vi "Convert Material JSON to LabVIEW Theme.vi"() -> ()   [LabVIEW 2021]
doc: "Convert existing material3 json files exported from Google to be used with TSC Material application VIs.\n\n<b>Code Developed By:</b>\nDaniel Coons\nTechnology Service Corporation\nwww.tsc.com/atcs"
uses:
  Material Theme/Material Theme.lvclass
  <vilib>/Utility/traverseref.llb/TRef TravTarget.ctl
  _Material Theme SubVIs/material theme.ctl
  _Material Theme SubVIs/material json scheme.ctl
  _Material Theme SubVIs/material json palette.ctl
  Material-Scheme/Material-Scheme.lvclass/Material-Scheme.ctl
  8aff6bdd-0f42-4725-a4f4-6aecb987c99b.vi
  Material-Scheme/data member access/get surface.vi
  Material-Scheme/data member access/Read name.vi
  <vilib>/JDP Science/JSONtext/JSON text to Variant.vi
  <vilib>/JDP Science/JSONtext/LVClass Serializer/JSONtext LVClass Serializer.lvclass
  Material-Palette/Material-Palette.lvclass
  Material-Scheme/Material-Scheme.lvclass
  user32.dll
  <vilib>/Utility/traverseref.llb/VI Scripting - Traverse.lvlib
panel:
  in  "tabs":enum32{"color", "palette", "json"}(radio)
  in  "preview":bool
  in  "close":bool
  out "header":bool
  in  "save":bool
  in  "Theme":u16(ring) items=["Light Theme", "Light Medium Contrast", "Light High Contrast", "Dark Theme", "Dark Medium Contrast", "Dark High Constrast"]
  in  "Tab Control":T1(tab)
  out "material JSON output":string
  in  "file path":path
  # "Convert a JSON M3 theme file from Google to use the TSC Material Theme in a VI"
  # "Can be generated through Figma or at:   https://material-foundation.github.io/material-theme-builder/<Material Website>"
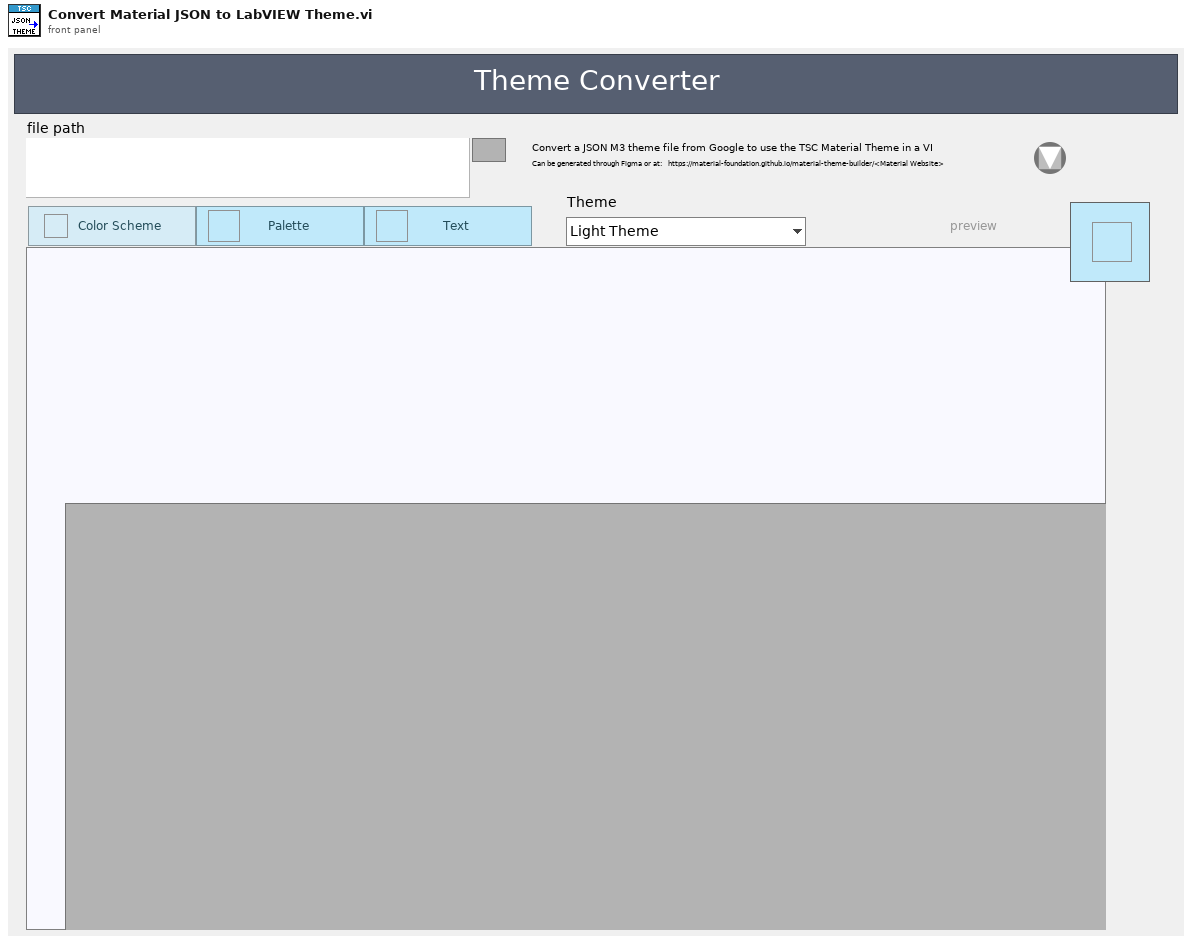
[diagram p1: front panel]
types:
  T1 = enum32{"Color Scheme", "Palette Variations", "JSON String"}
  T2 = typedef "TRef TravTarget.ctl" = enum16{"FP", "BD", "Other"}
  T3 = typedef "material theme.ctl" = cluster{"description":string, "seed":string, "coreColors":cluster{"primary":string, "secondary":string, "tertiary":string, "error":string}, "schemes":cluster{"light":T4, "light-medium-contrast":T4, "light-high-contrast":T4, "dark":T4, "dark-medium-contrast":T4, "dark-high-contrast":T4}, "palettes":cluster{"primary":T5, "secondary":T5, "tertiary":T5, "neutral":T5, "neutral-variant":T5}}
  T4 = typedef "material json scheme.ctl" = cluster{"primary":string, "surfaceTint":string, "onPrimary":string, "primaryContainer":string, "onPrimaryContainer":string, "secondary":string, "onSecondary":string, "secondaryContainer":string, "onSecondaryContainer":string, "tertiary":string, "onTertiary":string, "tertiaryContainer":string, "onTertiaryContainer":string, "error":string, "onError":string, "errorContainer":string, "onErrorContainer":string, "background":string, "onBackground":string, "surface":string, "onSurface":string, "surfaceVariant":string, "onSurfaceVariant":string, "outline":string, "outlineVariant":string, "shadow":string, "scrim":string, "inverseSurface":string, "inverseOnSurface":string, "inversePrimary":string, "primaryFixed":string, "onPrimaryFixed":string, "primaryFixedDim":string, "onPrimaryFixedVariant":string, "secondaryFixed":string, "onSecondaryFixed":string, "secondaryFixedDim":string, "onSecondaryFixedVariant":string, "tertiaryFixed":string, "onTertiaryFixed":string, "tertiaryFixedDim":string, "onTertiaryFixedVariant":string, "surfaceDim":string, "surfaceBright":string, "surfaceContainerLowest":string, "surfaceContainerLow":string, "surfaceContainer":string, "surfaceContainerHigh":string, "surfaceContainerHighest":string}
  T5 = typedef "material json palette.ctl" = cluster{"0":string, "5":string, "10":string, "15":string, "20":string, "25":string, "30":string, "35":string, "40":string, "50":string, "60":string, "70":string, "80":string, "90":string, "95":string, "98":string, "99":string, "100":string}
  T6 = enum16{"open", "replace", "create", "open or create", "replace or create", "replace or create with confirmation"}
  T7 = typedef "LVRectTypeDef.ctl" = cluster{"Left":i16, "Top":i16, "Right":i16, "Bottom":i16}
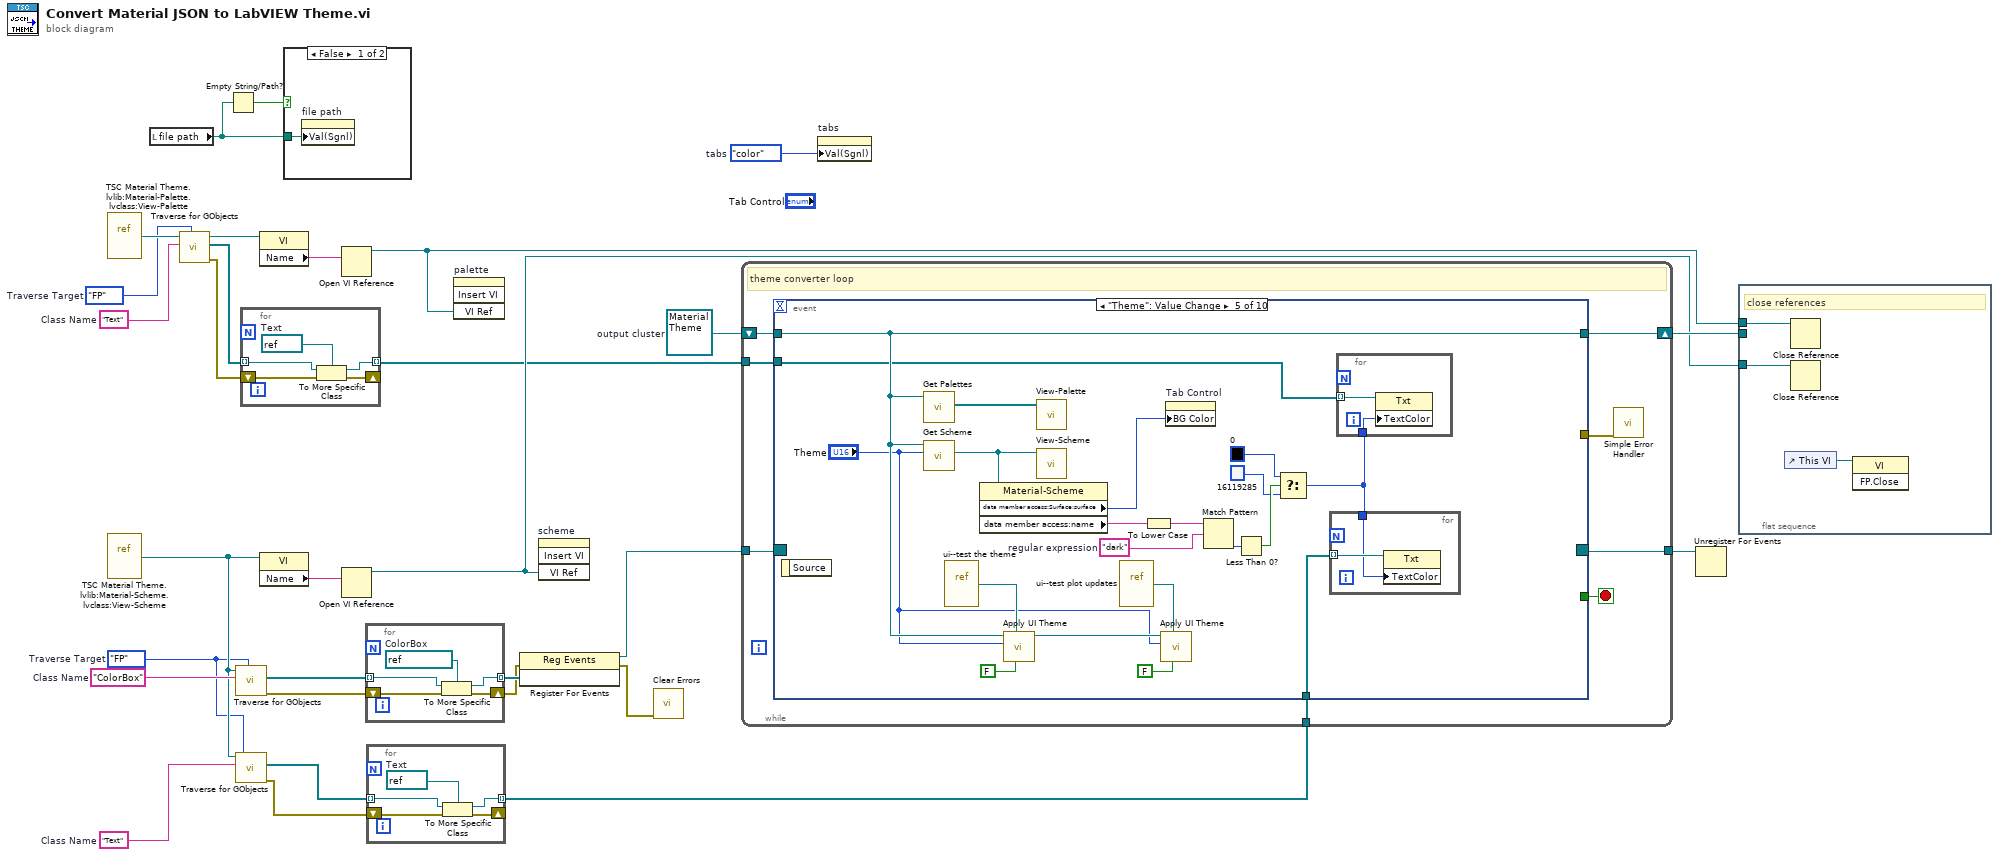
[diagram p0: block diagram]
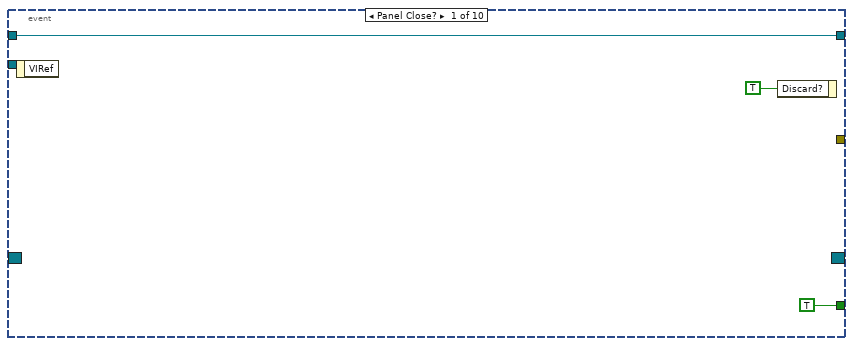
[diagram p3: hidden frame]
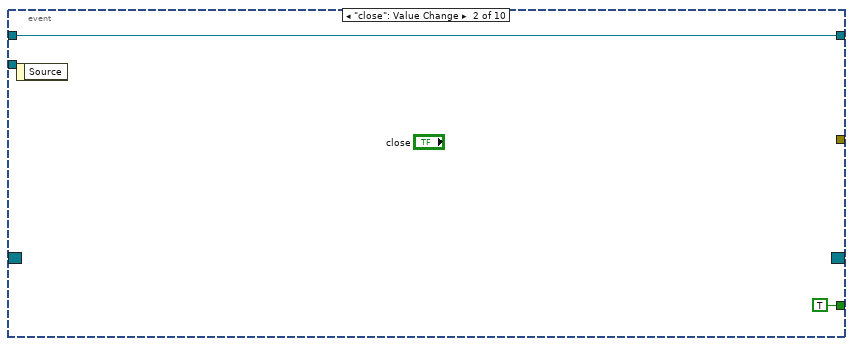
[diagram p4: hidden frame]
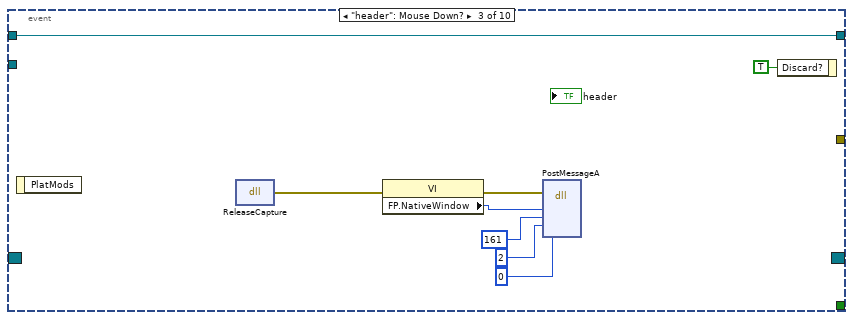
[diagram p5: hidden frame]
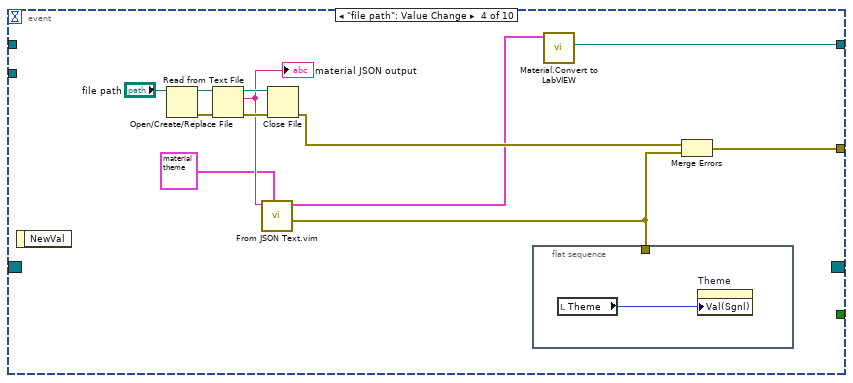
[diagram p6: hidden frame]
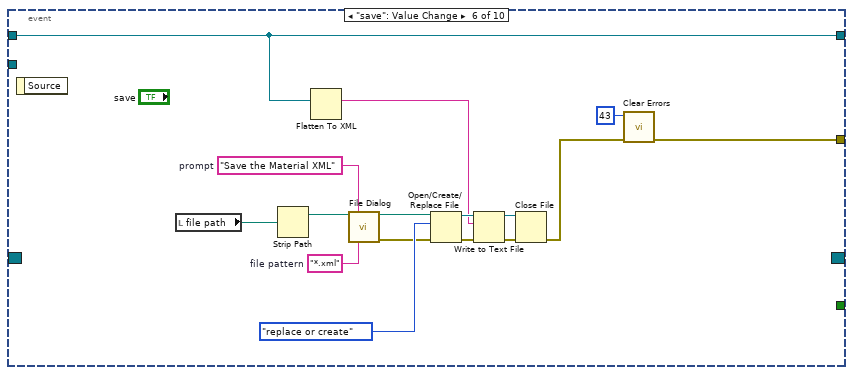
[diagram p7: hidden frame]
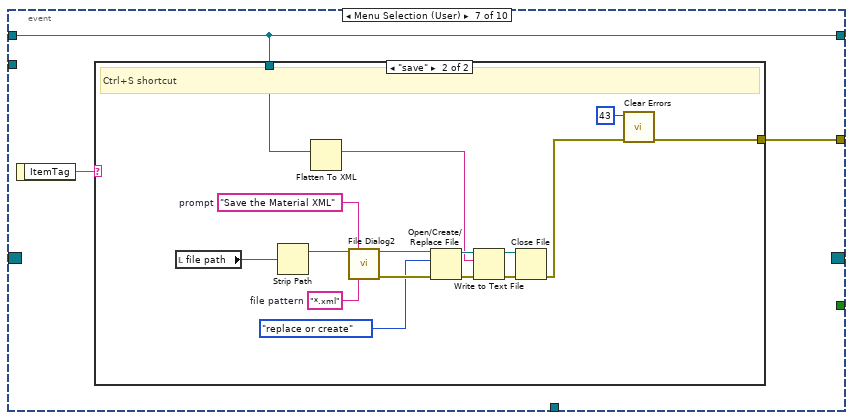
[diagram p8: hidden frame]
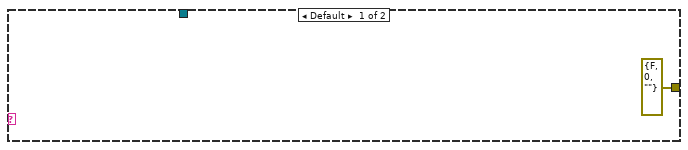
[diagram p9: hidden frame]
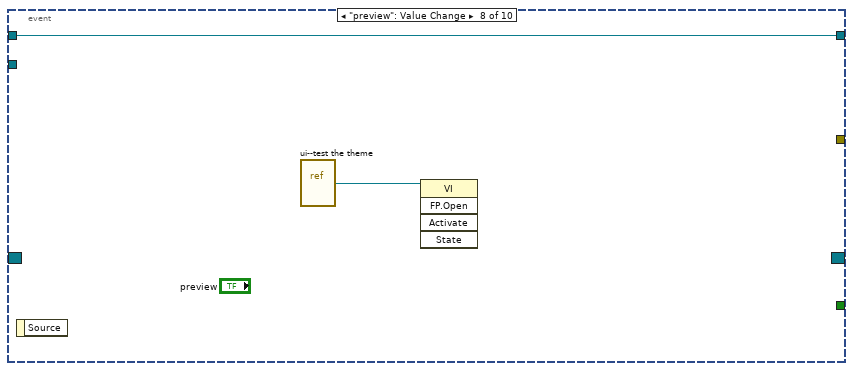
[diagram p10: hidden frame]
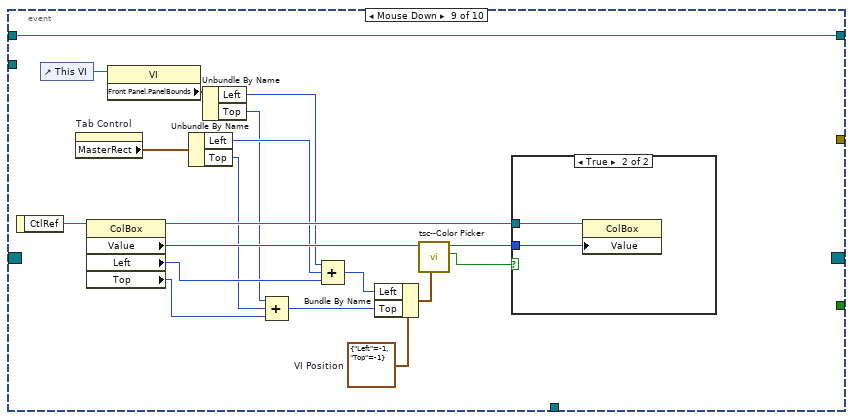
[diagram p11: hidden frame]
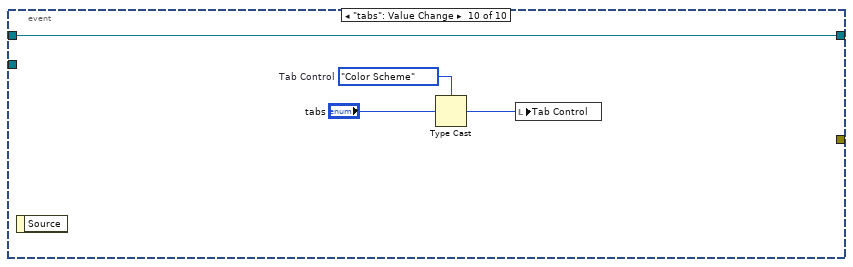
[diagram p13: hidden frame]
diagram:
  w6 = "Text"  # Class Name
  w10 = "Text"  # Class Name
  w11 = TRef_TravTarget."FP"  # Traverse Target
  w13 = enum32{"color", "palette", "json"}."color"  # tabs
  w16 = refnum<class "Material Theme.lvclass"> refnum  # output cluster
  w25 = "ColorBox"  # Class Name
  w4 = TRef_TravTarget."FP"  # Traverse Target
  n1 = vi-ref "TSC Material Theme.lvlib:Material-Palette.lvclass:View-Palette.vi"() -> (w30:refnum<vi>)
  n2 = vi-ref "TSC Material Theme.lvlib:Material-Scheme.lvclass:View-Scheme.vi"() -> (w5:refnum<vi>)
  n3 = local read "file path"() -> (w15:path)
  n4 = call <vilib>:"Traverse for GObjects.vi"("Traverse Target"=w11, "Class Name"=w10, "VI Refnum"=w30) -> ("error out"=w7:errorcluster, "References"=w9:refnum<vi>[], "dup VI Refnum"=w12:refnum<vi>)  [unwired: 5 in, 1 out]
  n5 = Empty String/Path?(string/path=w15) -> (empty?=w14:bool)
  n6 = call <vilib>:"Traverse for GObjects.vi"("Traverse Target"=w4, "Class Name"=w25, "VI Refnum"=w5) -> ("error out"=w19:errorcluster, "References"=w23:refnum<vi>[])  [unwired: 5 in, 2 out]
  n7 = call <vilib>:"Traverse for GObjects.vi"("Traverse Target"=w4, "Class Name"=w6, "VI Refnum"=w5) -> ("error out"=w2:errorcluster, "References"=w3:refnum<vi>[])  [unwired: 5 in, 2 out]
  n8 = for {
    tunnel: w9 -> [w32] mode=indexing
    shift-right: [w34] -> _
    shift-left: w7 -> [w35]
    tunnel: [w31] -> w8 mode=indexing
    w33 = refnum<vi> refnum  # Text
    n9 = To More Specific Class(target class=w33, reference=w32, error in=w35) -> (specific class reference=w31:refnum<vi>, error out=w34:errorcluster)
  }
  n10 = property class="VI"(reference=w12) -> ("Name"=w29:string)  [unwired: 1 in, 2 out]
  n11 = property class="VI"(reference=w5) -> ("Name"=w28:string)  [unwired: 1 in, 2 out]
  n12 = case shown="False" w14 {
    tunnel: w15 -> [w36 _]
    frame False {
      n13 = property on="file path" class="Path"("Val(Sgnl)"=w36) -> ()  [unwired: 2 in, 2 out]
    }
    frame True {
    }
  }
  n14 = Open VI Reference(vi path=w29) -> (vi reference=w26:refnum<vi>)  [unwired: 5 in, 1 out]
  n15 = Open VI Reference(vi path=w28) -> (vi reference=w22:refnum<vi>)  [unwired: 5 in, 1 out]
  n16 = for {
    tunnel: w23 -> [w38] mode=indexing
    shift-right: [w40] -> w18
    shift-left: w19 -> [w41]
    tunnel: [w37] -> w21 mode=indexing
    w39 = refnum<vi> refnum  # ColorBox
    n17 = To More Specific Class(target class=w39, reference=w38, error in=w41) -> (specific class reference=w37:refnum<vi>, error out=w40:errorcluster)
  }
  n18 = for {
    tunnel: w3 -> [w43] mode=indexing
    shift-right: [w45] -> _
    shift-left: w2 -> [w46]
    tunnel: [w42] -> w1 mode=indexing
    w44 = refnum<vi> refnum  # Text
    n19 = To More Specific Class(target class=w44, reference=w43, error in=w46) -> (specific class reference=w42:refnum<vi>, error out=w45:errorcluster)
  }
  n20 = invoke on="palette" class="SubPnl" method="Insert VI"("VI Ref"=w26) -> ()  [unwired: 3 in, 4 out]
  n21 = register-events(error in=w18, w21) -> (reference out=w24:refnum<event-registration>, error out=w17:errorcluster)  [unwired: 1 in]
  n22 = invoke on="scheme" class="SubPnl" method="Insert VI"("VI Ref"=w22) -> ()  [unwired: 3 in, 4 out]
  n23 = call <vilib>:"Clear Errors.vi"("error in (no error)"=w17) -> ()  [unwired: 5 in, 2 out]
  n24 = while {
    shift-right: [w53] -> w27
    shift-left: w16 -> [w52]
    tunnel: w24 -> [w50]
    tunnel: [w49] -> w20
    tunnel: w8 -> [w48]
    tunnel: w1 -> [w47]
    stop <- w54 stop-if-true
    # "theme converter loop"
    n25 = event shown="[4] \"Theme\": Value Change" {
      selector: w50 -> [_ _ _ _ _ _ _ _ _ _]
      dyn-events: [_ _ _ _ _ _ _ _ _ _] -> w49
      timeout: _ -> [_ _ _ _ _ _ _ _ _ _]
      tunnel: [TRUE TRUE _ _ _ _ _ _ _ _] -> w54
      tunnel: [w55 w59 w60 w74 w97 w114 w123 w142 w161 w167] -> w53
      tunnel: w52 -> [w55 w59 w60 _ w97 w114 w123 w142 w161 w167]
      tunnel: [_ _ _ w72 _ w112 w122 _ _ _] -> w51
      tunnel: w48 -> [_ _ _ _ w86 _ _ _ _ _]
      tunnel: w47 -> [_ _ _ _ w82 _ _ _ _ _]
      event Panel Close? {
        n26 = event-data() -> ()  [unwired: 1 in, 1 out]
        n27 = event-data("Discard?"=TRUE) -> ()  [unwired: 1 in, 1 out]
      }
      event "close": Value Change {
        n28 = event-data() -> ()  [unwired: 1 in, 1 out]
      }
      event "header": Mouse Down? {
        n29 = event-data() -> ()  [unwired: 1 in, 1 out]
        n30 = dll-call lib="user32.dll" fn="ReleaseCapture"() -> (error out=w63:errorcluster)  [unwired: 4 in, 1 out]
        n31 = property class="VI"(error in=w63) -> (error out=w62:errorcluster, "FP.NativeWindow"=w61:u64)  [unwired: 1 in, 1 out]
        n32 = dll-call lib="user32.dll" fn="PostMessageA"(error in=w62, "hWnd"=w61, "Msg"=161, "wParam"=2, "lParam"=0) -> ()  [unwired: 7 in, 2 out]
        n33 = event-data("Discard?"=TRUE) -> ()  [unwired: 1 in, 1 out]
      }
      event "file path": Value Change {
        n34 = event-data() -> ()  [unwired: 1 in, 1 out]
        n35 = Open/Create/Replace File(file path (use dialog)="file path") -> (refnum out=w75:refnum<file>, error out=w76:errorcluster)  [unwired: 5 in, 1 out]
        n36 = Read from Text File(file (use dialog)=w75, error in=w76) -> (refnum out=w77:refnum<file>, text=w71:string, error out=w78:errorcluster)  [unwired: 2 in, 1 out]
        "material JSON output" <- w71
        n37 = call "From JSON Text.vim"("Data Type and Default Value"=T3 {"description"="", "seed"="", "coreColors"={"primary"="", "secondary"="", "tertiary"="", "error"=""}, "schemes"={"light"={"primary"="", "surfaceTint"="", "onPrimary"="", "primaryContainer"="0", "onPrimaryContainer"="0", "secondary"="0", "onSecondary"="0", "secondaryContainer"="0", "onSecondaryContainer"="0", "tertiary"="0", "onTertiary"="0", "tertiaryContainer"="0", "onTertiaryContainer"="0", "error"="0", "onError"="0", "errorContainer"="0", "onErrorContainer"="0", "background"="0", "onBackground"="0", "surface"="0", "onSurface"="0", "surfaceVariant"="0", "onSurfaceVariant"="0", "outline"="0", "outlineVariant"="0", "shadow"="0", "scrim"="0", "inverseSurface"="0", "inverseOnSurface"="0", "inversePrimary"="", "primaryFixed"="0", "onPrimaryFixed"="0", "primaryFixedDim"="0", "onPrimaryFixedVariant"="0", "secondaryFixed"="0", "onSecondaryFixed"="0", "secondaryFixedDim"="0", "onSecondaryFixedVariant"="0", "tertiaryFixed"="0", "onTertiaryFixed"="0", "tertiaryFixedDim"="0", "onTertiaryFixedVariant"="0", "surfaceDim"="0", "surfaceBright"="0", "surfaceContainerLowest"="0", "surfaceContainerLow"="0", "surfaceContainer"="0", "surfaceContainerHigh"="0", "surfaceContainerHighest"="0"}, "light-medium-contrast"={"primary"="", "surfaceTint"="", "onPrimary"="", "primaryContainer"="0", "onPrimaryContainer"="0", "secondary"="0", "onSecondary"="0", "secondaryContainer"="0", "onSecondaryContainer"="0", "tertiary"="0", "onTertiary"="0", "tertiaryContainer"="0", "onTertiaryContainer"="0", "error"="0", "onError"="0", "errorContainer"="0", "onErrorContainer"="0", "background"="0", "onBackground"="0", "surface"="0", "onSurface"="0", "surfaceVariant"="0", "onSurfaceVariant"="0", "outline"="0", "outlineVariant"="0", "shadow"="0", "scrim"="0", "inverseSurface"="0", "inverseOnSurface"="0", "inversePrimary"="", "primaryFixed"="0", "onPrimaryFixed"="0", "primaryFixedDim"="0", "onPrimaryFixedVariant"="0", "secondaryFixed"="0", "onSecondaryFixed"="0", "secondaryFixedDim"="0", "onSecondaryFixedVariant"="0", "tertiaryFixed"="0", "onTertiaryFixed"="0", "tertiaryFixedDim"="0", "onTertiaryFixedVariant"="0", "surfaceDim"="0", "surfaceBright"="0", "surfaceContainerLowest"="0", "surfaceContainerLow"="0", "surfaceContainer"="0", "surfaceContainerHigh"="0", "surfaceContainerHighest"="0"}, "light-high-contrast"={"primary"="", "surfaceTint"="", "onPrimary"="", "primaryContainer"="0", "onPrimaryContainer"="0", "secondary"="0", "onSecondary"="0", "secondaryContainer"="0", "onSecondaryContainer"="0", "tertiary"="0", "onTertiary"="0", "tertiaryContainer"="0", "onTertiaryContainer"="0", "error"="0", "onError"="0", "errorContainer"="0", "onErrorContainer"="0", "background"="0", "onBackground"="0", "surface"="0", "onSurface"="0", "surfaceVariant"="0", "onSurfaceVariant"="0", "outline"="0", "outlineVariant"="0", "shadow"="0", "scrim"="0", "inverseSurface"="0", "inverseOnSurface"="0", "inversePrimary"="", "primaryFixed"="0", "onPrimaryFixed"="0", "primaryFixedDim"="0", "onPrimaryFixedVariant"="0", "secondaryFixed"="0", "onSecondaryFixed"="0", "secondaryFixedDim"="0", "onSecondaryFixedVariant"="0", "tertiaryFixed"="0", "onTertiaryFixed"="0", "tertiaryFixedDim"="0", "onTertiaryFixedVariant"="0", "surfaceDim"="0", "surfaceBright"="0", "surfaceContainerLowest"="0", "surfaceContainerLow"="0", "surfaceContainer"="0", "surfaceContainerHigh"="0", "surfaceContainerHighest"="0"}, "dark"={"primary"="", "surfaceTint"="", "onPrimary"="", "primaryContainer"="0", "onPrimaryContainer"="0", "secondary"="0", "onSecondary"="0", "secondaryContainer"="0", "onSecondaryContainer"="0", "tertiary"="0", "onTertiary"="0", "tertiaryContainer"="0", "onTertiaryContainer"="0", "error"="0", "onError"="0", "errorContainer"="0", "onErrorContainer"="0", "background"="0", "onBackground"="0", "surface"="0", "onSurface"="0", "surfaceVariant"="0", "onSurfaceVariant"="0", "outline"="0", "outlineVariant"="0", "shadow"="0", "scrim"="0", "inverseSurface"="0", "inverseOnSurface"="0", "inversePrimary"="", "primaryFixed"="0", "onPrimaryFixed"="0", "primaryFixedDim"="0", "onPrimaryFixedVariant"="0", "secondaryFixed"="0", "onSecondaryFixed"="0", "secondaryFixedDim"="0", "onSecondaryFixedVariant"="0", "tertiaryFixed"="0", "onTertiaryFixed"="0", "tertiaryFixedDim"="0", "onTertiaryFixedVariant"="0", "surfaceDim"="0", "surfaceBright"="0", "surfaceContainerLowest"="0", "surfaceContainerLow"="0", "surfaceContainer"="0", "surfaceContainerHigh"="0", "surfaceContainerHighest"="0"}, "dark-medium-contrast"={"primary"="", "surfaceTint"="", "onPrimary"="", "primaryContainer"="0", "onPrimaryContainer"="0", "secondary"="0", "onSecondary"="0", "secondaryContainer"="0", "onSecondaryContainer"="0", "tertiary"="0", "onTertiary"="0", "tertiaryContainer"="0", "onTertiaryContainer"="0", "error"="0", "onError"="0", "errorContainer"="0", "onErrorContainer"="0", "background"="0", "onBackground"="0", "surface"="0", "onSurface"="0", "surfaceVariant"="0", "onSurfaceVariant"="0", "outline"="0", "outlineVariant"="0", "shadow"="0", "scrim"="0", "inverseSurface"="0", "inverseOnSurface"="0", "inversePrimary"="", "primaryFixed"="0", "onPrimaryFixed"="0", "primaryFixedDim"="0", "onPrimaryFixedVariant"="0", "secondaryFixed"="0", "onSecondaryFixed"="0", "secondaryFixedDim"="0", "onSecondaryFixedVariant"="0", "tertiaryFixed"="0", "onTertiaryFixed"="0", "tertiaryFixedDim"="0", "onTertiaryFixedVariant"="0", "surfaceDim"="0", "surfaceBright"="0", "surfaceContainerLowest"="0", "surfaceContainerLow"="0", "surfaceContainer"="0", "surfaceContainerHigh"="0", "surfaceContainerHighest"="0"}, "dark-high-contrast"={"primary"="", "surfaceTint"="", "onPrimary"="", "primaryContainer"="0", "onPrimaryContainer"="0", "secondary"="0", "onSecondary"="0", "secondaryContainer"="0", "onSecondaryContainer"="0", "tertiary"="0", "onTertiary"="0", "tertiaryContainer"="0", "onTertiaryContainer"="0", "error"="0", "onError"="0", "errorContainer"="0", "onErrorContainer"="0", "background"="0", "onBackground"="0", "surface"="0", "onSurface"="0", "surfaceVariant"="0", "onSurfaceVariant"="0", "outline"="0", "outlineVariant"="0", "shadow"="0", "scrim"="0", "inverseSurface"="0", "inverseOnSurface"="0", "inversePrimary"="", "primaryFixed"="0", "onPrimaryFixed"="0", "primaryFixedDim"="0", "onPrimaryFixedVariant"="0", "secondaryFixed"="0", "onSecondaryFixed"="0", "secondaryFixedDim"="0", "onSecondaryFixedVariant"="0", "tertiaryFixed"="0", "onTertiaryFixed"="0", "tertiaryFixedDim"="0", "onTertiaryFixedVariant"="0", "surfaceDim"="0", "surfaceBright"="0", "surfaceContainerLowest"="0", "surfaceContainerLow"="0", "surfaceContainer"="0", "surfaceContainerHigh"="0", "surfaceContainerHighest"="0"}}, "palettes"={"primary"={"0"="0", "5"="0", "10"="0", "15"="0", "20"="0", "25"="0", "30"="0", "35"="0", "40"="0", "50"="0", "60"="0", "70"="0", "80"="0", "90"="0", "95"="0", "98"="0", "99"="0", "100"="0"}, "secondary"={"0"="0", "5"="0", "10"="0", "15"="0", "20"="0", "25"="0", "30"="0", "35"="0", "40"="0", "50"="0", "60"="0", "70"="0", "80"="0", "90"="0", "95"="0", "98"="0", "99"="0", "100"="0"}, "tertiary"={"0"="0", "5"="0", "10"="0", "15"="0", "20"="0", "25"="0", "30"="0", "35"="0", "40"="0", "50"="0", "60"="0", "70"="0", "80"="0", "90"="0", "95"="0", "98"="0", "99"="0", "100"="0"}, "neutral"={"0"="0", "5"="0", "10"="0", "15"="0", "20"="0", "25"="0", "30"="0", "35"="0", "40"="0", "50"="0", "60"="0", "70"="0", "80"="0", "90"="0", "95"="0", "98"="0", "99"="0", "100"="0"}, "neutral-variant"={"0"="0", "5"="0", "10"="0", "15"="0", "20"="0", "25"="0", "30"="0", "35"="0", "40"="0", "50"="0", "60"="0", "70"="0", "80"="0", "90"="0", "95"="0", "98"="0", "99"="0", "100"="0"}}}, "JSON"=w71) -> ("error out"=w70:errorcluster, "Data out"=w68:T3)  [unwired: 8 in]
        n38 = Close File(refnum=w77, error in=w78) -> (error out=w73:errorcluster)  [unwired: 1 out]
        n39 = flat-sequence {
          tunnel: w70 -> [_]
          frame #0 {
            n40 = local read "Theme"() -> (w80:u16)
            n41 = property on="Theme" class="Ring (strict)"("Val(Sgnl)"=w80) -> ()  [unwired: 2 in, 2 out]
          }
        }
        n42 = call "Material.Convert to LabVIEW.vi"("material.json string"=w68) -> ("output cluster"=w74:refnum<class "Material Theme.lvclass">)  [unwired: 10 in]
        n43 = Merge Errors(w73, w70) -> (w72:errorcluster)
      }
      event "Theme": Value Change {
        w89 = "dark"  # regular expression
        n44 = event-data() -> ()  [unwired: 1 in, 1 out]
        n45 = call "Get Palettes.vi"("Material Theme in"=w97) -> ("Material-Scheme"=w100:refnum<class "Material-Palette.lvclass">[])  [unwired: 8 in, 2 out]
        n46 = call "Get Scheme.vi"("Theme"="Theme", "Material Theme in"=w97) -> ("Material-Scheme"=w92:refnum<class "Material-Scheme.lvclass">)  [unwired: 7 in, 2 out]
        n47 = vi-ref "ui--test the theme.vi"() -> (w99:refnum<vi>)
        n48 = property class="Material-Scheme"(reference=w92) -> ("data member access:Surface:surface"=w91:u32, "data member access:name"=w90:string)  [unwired: 1 in, 2 out]
        n49 = call "Apply UI Theme.vi"("save?"=FALSE, "VI Refnum"=w99, "Theme"="Theme", "Material Theme in"=w97) -> ("Material Theme out"=w95:refnum<class "Material Theme.lvclass">)  [unwired: 6 in, 1 out]
        n50 = call "View-Palette.vi"("Array"=w100) -> ()  [unwired: 11 in]
        n51 = call "View-Scheme.vi"("Material-Scheme.lvclass"=w92) -> ()  [unwired: 11 in]
        n52 = vi-ref "ui--test plot updates.vi"() -> (w96:refnum<vi>)
        n53 = To Lower Case(string=w90) -> (all lower case string=w88:string)
        n54 = call "Apply UI Theme.vi"("save?"=FALSE, "VI Refnum"=w96, "Theme"="Theme", "Material Theme in"=w95) -> ()  [unwired: 6 in, 2 out]
        n55 = property on="Tab Control" class="TabCtl (strict)"("BG Color"=w91) -> ()  [unwired: 2 in, 2 out]
        n56 = Match Pattern(string=w88, regular expression=w89) -> (offset past match=w87:i32)  [unwired: 1 in, 3 out]
        n57 = Less Than 0?(x=w87) -> (x < 0?=w85:bool)
        n58 = Select(t=u32 0, s=w85, f=u32 16119285) -> (s? t:f=w81:u32)
        n59 = for {
          tunnel: w82 -> [w102] mode=indexing
          tunnel: w81 -> [w101]
          n60 = property on="Property Node" class="Txt"(reference=w102, "TextColor"=w101) -> ()  [unwired: 1 in, 2 out]
        }
        n61 = for {
          tunnel: w86 -> [w104] mode=indexing
          tunnel: w81 -> [w103]
          n62 = property on="Property Node" class="Txt"(reference=w104, "TextColor"=w103) -> ()  [unwired: 1 in, 2 out]
        }
      }
      event "save": Value Change {
        w105 = "Save the Material XML"  # prompt
        w108 = "*.xml"  # file pattern
        n63 = event-data() -> ()  [unwired: 1 in, 1 out]
        n64 = local read "file path"() -> (w107:path)
        n65 = Strip Path(path=w107) -> (stripped path=w106:path)  [unwired: 1 out]
        n66 = Flatten To XML(6:w114) -> (2:w113:string)
        n67 = call "File Dialog"("start path"=w106, "prompt"=w105, "pattern (all files)"=w108) -> ("selected path"=w109:path, "error out"=w110:errorcluster)  [unwired: 9 in, 2 out]
        n68 = Open/Create/Replace File(file path (use dialog)=w109, error in=w110, operation (0:open)=T6."replace or create") -> (refnum out=w117:refnum<file>, error out=w119:errorcluster)  [unwired: 3 in, 1 out]
        n69 = Write to Text File(file (use dialog)=w117, text=w113, error in=w119) -> (refnum out=w116:refnum<file>, error out=w120:errorcluster)  [unwired: 1 in, 1 out]
        n70 = Close File(refnum=w116, error in=w120) -> (error out=w115:errorcluster)  [unwired: 1 out]
        n71 = call <vilib>:"Clear Errors.vi"("error in (no error)"=w115, "specific error code to clear (0: all)"=43) -> ("error out"=w112:errorcluster)  [unwired: 4 in, 1 out]
      }
      event Menu Selection (User) {
        n72 = event-data() -> ("ItemTag"=w121:string)  [unwired: 1 in]
        n73 = case shown="\"save\"" w121 {
          tunnel: w123 -> [_ w140]
          tunnel: [errorcluster {"status"=FALSE, "code"=0, "source"=""} ("error out") w139] -> w122
          frame Default {
          }
          frame "save" {
            w129 = "Save the Material XML"  # prompt
            w128 = "*.xml"  # file pattern
            # "Ctrl+S shortcut"
            n74 = local read "file path"() -> (w131:path)
            n75 = Strip Path(path=w131) -> (stripped path=w130:path)  [unwired: 1 out]
            n76 = Flatten To XML(6:w140) -> (2:w126:string)
            n77 = call "File Dialog2"("start path"=w130, "prompt"=w129, "pattern (all files)"=w128) -> ("selected path"=w132:path, "error out"=w133:errorcluster)  [unwired: 9 in, 2 out]
            n78 = Open/Create/Replace File(file path (use dialog)=w132, error in=w133, operation (0:open)=T6."replace or create") -> (refnum out=w135:refnum<file>, error out=w136:errorcluster)  [unwired: 3 in, 1 out]
            n79 = Write to Text File(file (use dialog)=w135, text=w126, error in=w136) -> (refnum out=w134:refnum<file>, error out=w137:errorcluster)  [unwired: 1 in, 1 out]
            n80 = Close File(refnum=w134, error in=w137) -> (error out=w125:errorcluster)  [unwired: 1 out]
            n81 = call <vilib>:"Clear Errors.vi"("error in (no error)"=w125, "specific error code to clear (0: all)"=43) -> ("error out"=w139:errorcluster)  [unwired: 4 in, 1 out]
          }
        }
      }
      event "preview": Value Change {
        n82 = event-data() -> ()  [unwired: 1 in, 1 out]
        n83 = vi-ref "ui--test the theme.vi"() -> (w141:refnum<vi>)
        n84 = invoke class="VI" method="FP.Open"(reference=w141) -> ()  [unwired: 4 in, 5 out]
      }
      event Mouse Down {
        w155 = cluster{"Left":i16, "Top":i16} {"Left"=-1, "Top"=-1}  # VI Position
        n85 = event-data() -> ("CtlRef"=w160:refnum<vi>)  [unwired: 1 in]
        n86 = control-ref of="This VI"() -> (w147:refnum<vi>)
        n87 = property on="Tab Control" class="TabCtl (strict)"() -> ("MasterRect"=w150:T7)  [unwired: 2 in, 2 out]
        n88 = property class="ColBox"(reference=w160) -> (reference out=w159:refnum<vi>, "Value"=w158:u32, "Left"=w152:i32, "Top"=w151:i32)  [unwired: 1 in, 1 out]
        n89 = property class="VI"(reference=w147) -> ("Front Panel.PanelBounds"=w146:T7)  [unwired: 1 in, 2 out]
        n90 = Unbundle By Name(w150) -> ("Left"=w149:i16, "Top"=w148:i16)
        n91 = Unbundle By Name(w146) -> ("Left"=w145:i16, "Top"=w144:i16)
        n92 = Compound Arithmetic op=ADD(w144, w148, w151) -> (w143:i32)
        n93 = Compound Arithmetic op=ADD(w145, w149, w152) -> (w153:i32)
        n94 = Bundle By Name(cluster=w155, "Left"=w153, "Top"=w143) -> (w154:cluster{"Left":i16, "Top":i16})
        n95 = call "tsc--Color Picker.vi"("VI Position"=w154, "input"=w158) -> ("accepted?"=w156:bool, "Resolved Color"=w157:u32)  [unwired: 8 in]
        n96 = case shown="True" w156 {
          tunnel: w157 -> [_ w163]
          tunnel: w159 -> [_ w162]
          frame False {
          }
          frame True {
            n97 = property class="ColBox"(reference=w162, "Value"=w163) -> ()  [unwired: 1 in, 2 out]
          }
        }
      }
      event "tabs": Value Change {
        w164 = T1."Color Scheme"  # Tab Control
        n98 = event-data() -> ()  [unwired: 1 in, 1 out]
        n99 = Type Cast(type=w164, x="tabs") -> (*(type *) &x=w165:T1)
        n100 = local write "Tab Control"(w165) -> ()
      }
    }
    n101 = call <vilib>:"Simple Error Handler.vi"("error in (no error)"=w51) -> ()  [unwired: 4 in, 5 out]
  }
  n102 = property on="tabs" class="RadioBtnsControl (strict)"("Val(Sgnl)"=w13) -> ()  [unwired: 2 in, 2 out]
  n103 = Unregister For Events(event registration refnum=w20) -> ()  [unwired: 1 in, 1 out]
  n104 = flat-sequence {
    tunnel: w27 -> [_]
    tunnel: w26 -> [w170]
    tunnel: w22 -> [w169]
    frame #0 {
      # "close references"
      n105 = control-ref of="This VI"() -> (w168:refnum<vi>)
      n106 = Close Reference(reference=w170) -> ()  [unwired: 1 in, 1 out]
      n107 = Close Reference(reference=w169) -> ()  [unwired: 1 in, 1 out]
      n108 = invoke class="VI" method="FP.Close"(reference=w168) -> ()  [unwired: 2 in, 3 out]
    }
  }
